vi "test refnum.vi"() -> ()   [LabVIEW 2010]
panel:
  out "algOutputMsgs 2":cluster{"MSG":i16, "Param":i32, "type":i16}[](array[cluster])
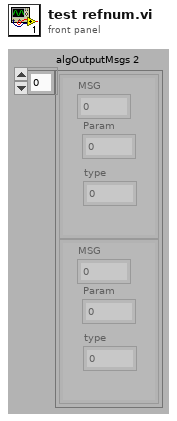
[diagram p1: front panel]
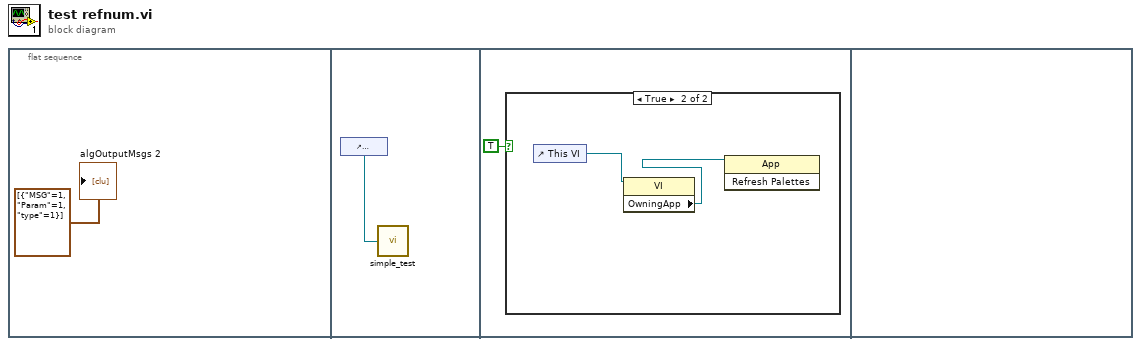
[diagram p0: block diagram]
diagram:
  n1 = flat-sequence {
    frame #0 {
      "algOutputMsgs 2" <- cluster{"MSG":i16, "Param":i32, "type":i16}[] [{"MSG"=1, "Param"=1, "type"=1}] ("algOutputMsgs 2")
    }
    frame #1 {
      n2 = control-ref of="algOutputMsgs 2"() -> (w2:refnum<vi>)
      n3 = call "simple_test.vi"("Arr Refnum"=w2) -> ()  [unwired: 1 in]
    }
    frame #2 {
      n4 = case shown="True" TRUE {
        frame False {
        }
        frame True {
          n5 = control-ref of="This VI"() -> (w5:refnum<vi>)
          n6 = property class="VI"(reference=w5) -> ("OwningApp"=w4:refnum<vi>)  [unwired: 1 in, 2 out]
          n7 = invoke class="App" method="Refresh Palettes"(reference=w4) -> ()  [unwired: 2 in, 3 out]
        }
      }
    }
    frame #3 {
    }
  }
